vi "prepareTestParameters.vi"(8 "error in (no error)":errorcluster, 11 "TestDataLog in":refnum<class "TestDataLog.lvclass">) -> (0 "error out":errorcluster, 2 "TestParameters":string, 3 "TestDataLog out":refnum<class "TestDataLog.lvclass">)   [LabVIEW 2013, in "TestDataLog.lvclass"]
uses:
  TestDataLog.lvclass
  TestDataLog.lvclass/TestDataLog.ctl
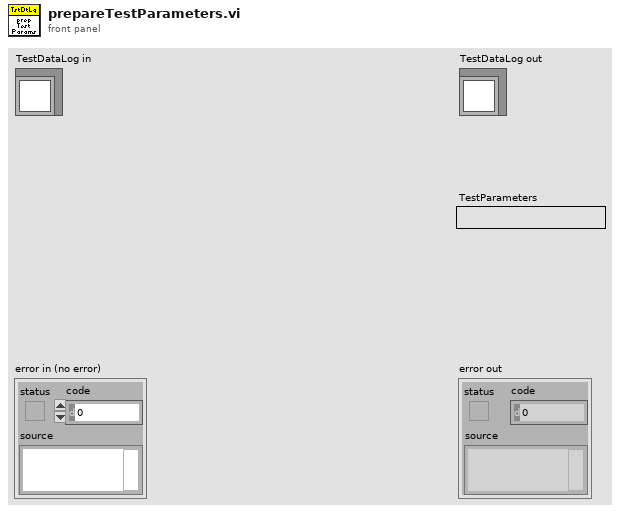
[diagram p1: front panel]
types:
  T1 = typedef "TestParameters.ctl" = cluster{"Number of cycles for complete test":u32, "Cycle profile":T2}
  T2 = typedef "CycleProfileConfig.ctl" = cluster{"Force Setpoint":dbl[unit][], "Pause After":dbl[unit][]}
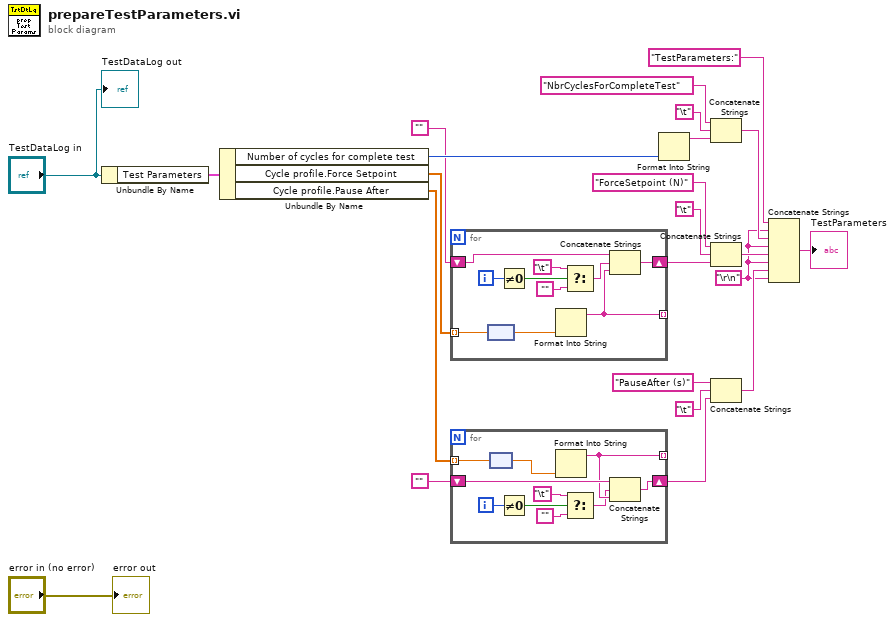
[diagram p0: block diagram]
diagram:
  w1 = "\r\n"
  n1 = Unbundle By Name("TestDataLog in") -> ("Test Parameters"=w22:T1)
  n2 = Unbundle By Name(w22) -> ("Number of cycles for complete test"=w21:u32, "Cycle profile.Force Setpoint"=w20:dbl[unit][], "Cycle profile.Pause After"=w18:dbl[unit][])
  n3 = for {
    tunnel: w20 -> [w28] mode=indexing
    shift-right: [w33] -> w9
    shift-left: "" -> [w32]
    tunnel: [w29] -> _ mode=indexing
    i -> [w31]
    n4 = node(w28) -> (w27:dbl)
    n5 = Not Equal To 0?(x=w31) -> (x != 0?=w30:bool)
    n6 = Format Into String(w27) -> (resulting string=w29:string)  [unwired: 3 in, 1 out]
    n7 = Select(t="\t", s=w30, f="") -> (s? t:f=w24:string)
    n8 = Concatenate Strings(w32, w24, w29) -> (w33:string)
  }
  n9 = for {
    tunnel: w18 -> [w38] mode=indexing
    shift-right: [w43] -> w5
    shift-left: "" -> [w42]
    tunnel: [w39] -> _ mode=indexing
    i -> [w41]
    n10 = node(w38) -> (w37:dbl)
    n11 = Not Equal To 0?(x=w41) -> (x != 0?=w40:bool)
    n12 = Format Into String(w37) -> (resulting string=w39:string)  [unwired: 3 in, 1 out]
    n13 = Select(t="\t", s=w40, f="") -> (s? t:f=w34:string)
    n14 = Concatenate Strings(w42, w34, w39) -> (w43:string)
  }
  n15 = Format Into String(w21) -> (resulting string=w12:string)  [unwired: 3 in, 1 out]
  n16 = Concatenate Strings("NbrCyclesForCompleteTest" ("element"), "\t", w12) -> (w14:string)
  n17 = Concatenate Strings("ForceSetpoint (N)" ("element"), "\t", w9) -> (w8:string)
  n18 = Concatenate Strings("PauseAfter (s)" ("element"), "\t", w5) -> (w4:string)
  n19 = Concatenate Strings("TestParameters:", w1, w14, w1, w8, w1, w4, w1) -> (→"TestParameters":string)
  "error out" <- "error in (no error)"
  "TestDataLog out" <- "TestDataLog in"
